vi "lv_Waveform.vi"() -> ()   [LabVIEW 2018]
panel:
  in  "位置参数":bool
  in  "时间模式":bool
  in  "还原指针":bool
  in  "鼠标拖动":bool
  in  "水平选择":bool
  in  "垂直选择":bool
  in  "点击缩小":bool
  in  "点击放大":bool
  in  "选择区域":bool
  in  "区域还原":bool
  in  "stop":bool
  out "Waveform Graph":waveform(dbl)(graph)
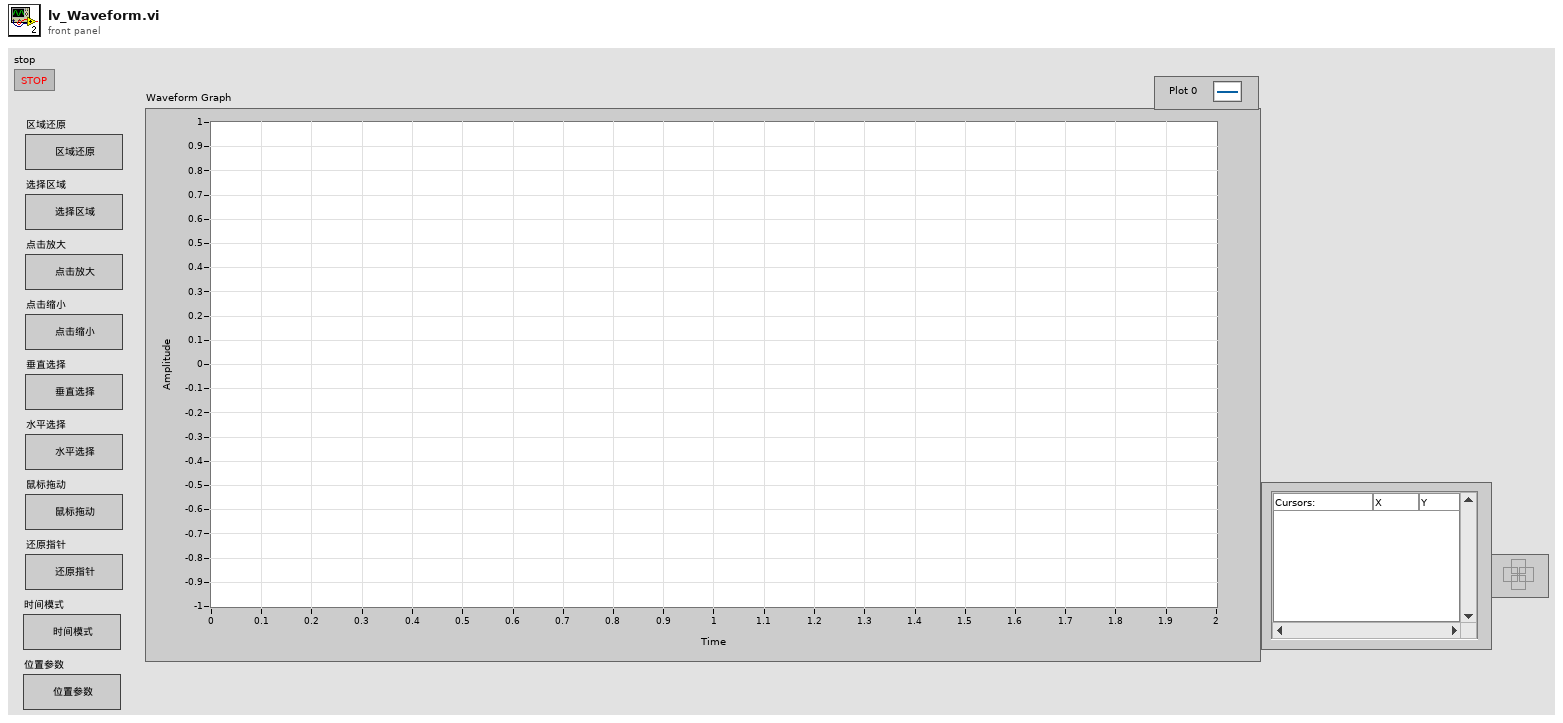
[diagram p1: front panel]
types:
  T1 = cluster{"Name":string, "Color":u32, "Style":u8, "Point Style":u8, "Name Visible":bool, "Allow Drag":bool, "Cursor Mode":u32, "Plot":i32, "Index":i32, "Position":cluster{"X":dbl, "Y":dbl}, "X Scale":u32, "Y Scale":u32, "Watch Plots":i32[], "Watch All Plots":bool, "Plot Area":i32, "Label Offset":cluster{"X":dbl, "Y":dbl}}
  T2 = cluster{"Boolean Text.Text":string, "Palette:Active Tool":i32}[]
  T3 = cluster{"Boolean Text.Text":string, "Palette:Active Tool":i32}
  T4 = typedef "LVPoint32TypeDef.ctl" = cluster{"Horizontal":i32, "Vertical":i32}
  T5 = typedef "LVCursorListTypeDef.ctl" = cluster{"Name":string, "Color":u32, "Style":u8, "Point Style":u8, "Name Visible":bool, "Allow Drag":bool, "Cursor Mode":u32, "Plot":i32, "Index":i32, "Position":cluster{"X":dbl, "Y":dbl}, "X Scale":u32, "Y Scale":u32, "Watch Plots":i32[], "Watch All Plots":bool, "Plot Area":i32, "Label Offset":cluster{"X":dbl, "Y":dbl}}[]
  T6 = typedef "LVRangeTypeDef.ctl" = cluster{"Minimum":dbl, "Maximum":dbl, "Increment":dbl, "Minor Increment":dbl, "Start":dbl}
  T7 = typedef "lveventtype.ctl" = enum32{"Null", "Timeout", "Annotation Menu Selection", "Annotation Menu Selection?", "App Instance Close", "App Instance Close?", "Autoscale Range Change", "Bookmark Info Change", "Cell Edit", "Cell Edit?", "Cursor Grab", "Cursor Grab?", "Cursor Menu Selection", "Cursor Menu Selection?", "Cursor Move", "Cursor Release", "Data Change", "Direction Change", "Display State Change", "Drag Ended", "Drag Enter", "Drag Leave", "Drag Over", "Drag Source Update", "Drag Starting", "Drag Starting?", "Drop", "Exec State Change", "Key Down", "Key Down?", "Key Repeat", "Key Repeat?", "Key Up", "Listbox Double Click", "Menu Activation?", "Menu Selection (App)", "Menu Selection? (App)", "Menu Selection (User)", "Mouse Down", "Mouse Down?", "Mouse Enter", "Mouse Leave", "Mouse Move", "Mouse Up", "Mouse Wheel", "NI Security User Change (App)", "Pane Size", "Panel Close", "Panel Close?", "Panel Resize", "Plot Attribute Change", "Scale Range Change", "Shortcut Menu Activation?", "Shortcut Menu Selection (App)", "Shortcut Menu Selection? (App)", "Shortcut Menu Selection (User)", "Tree Double Click", "Tree Drag", "Tree Drag?", "Tree Drop", "Tree Drop?", "Tree Item Close", "Tree Item Close?", "Tree Item Open", "Tree Item Open?", "User Event", "Value Change"}
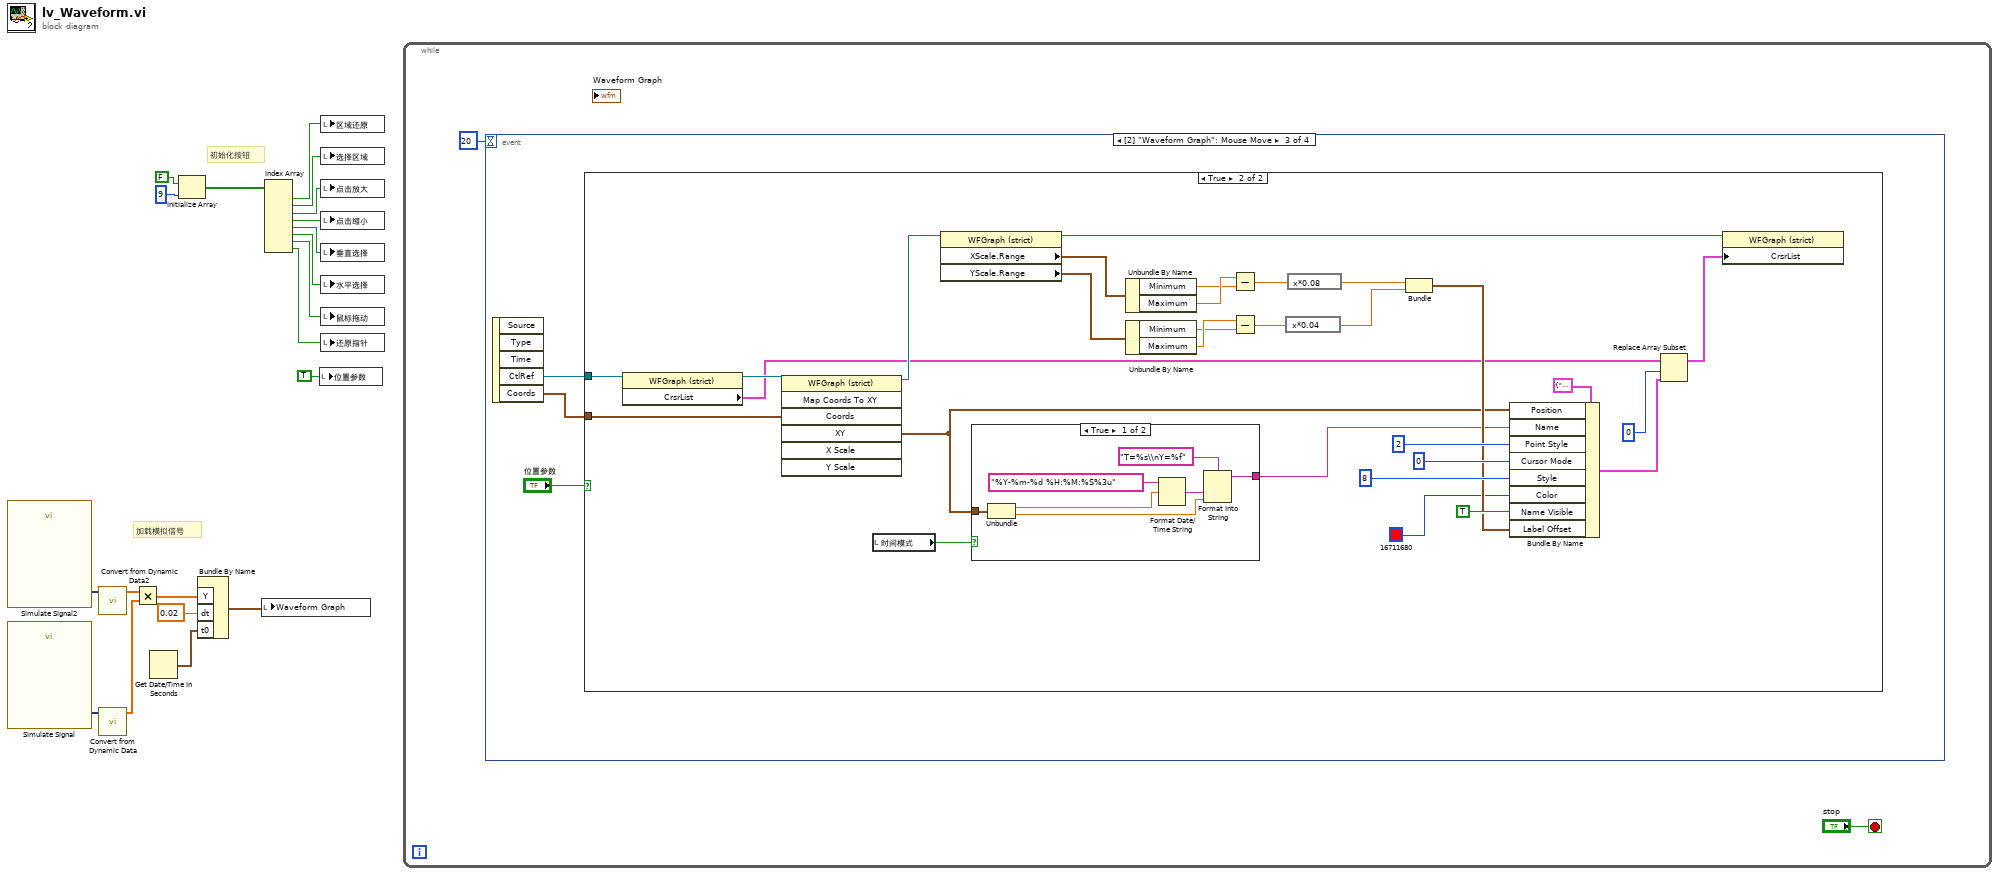
[diagram p0: block diagram]
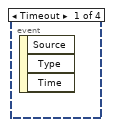
[diagram p2: hidden frame]
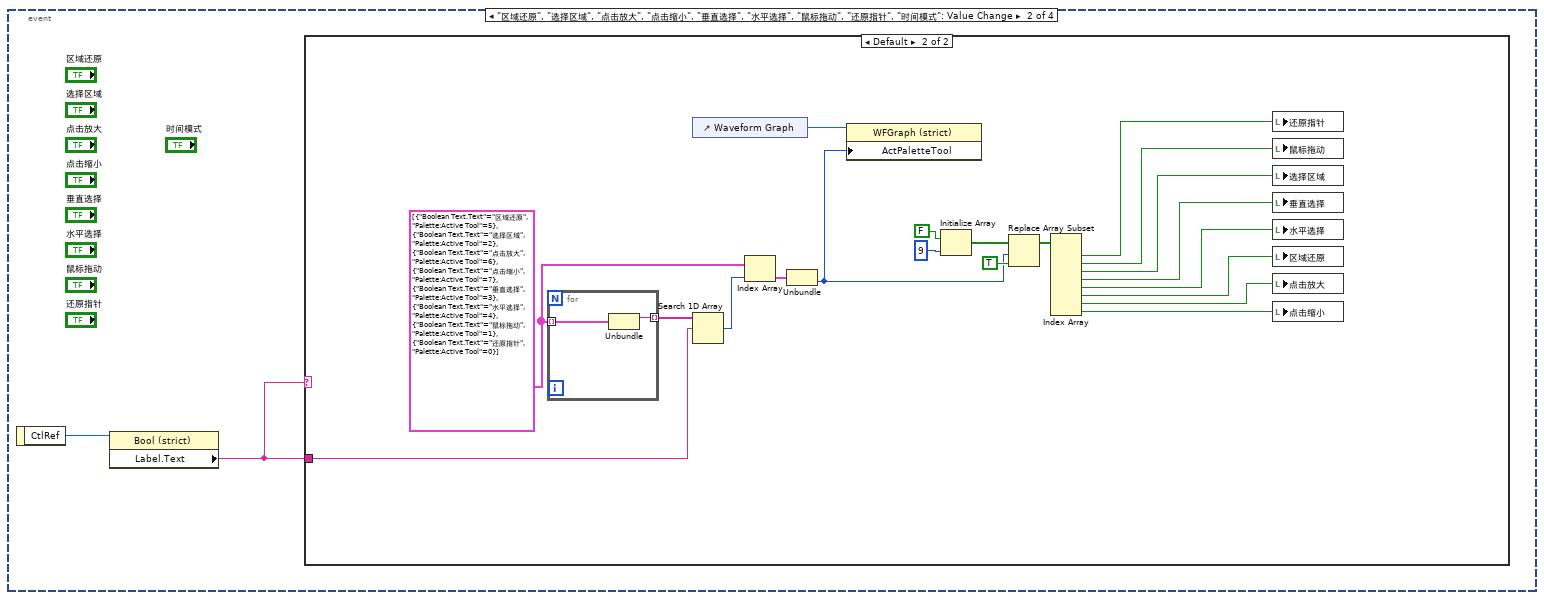
[diagram p3: hidden frame]
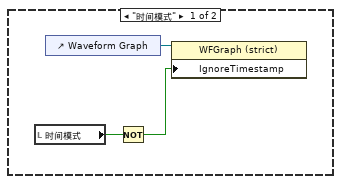
[diagram p4: hidden frame]
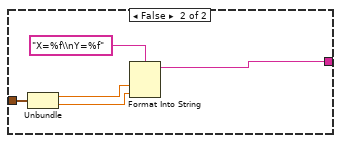
[diagram p6: hidden frame]
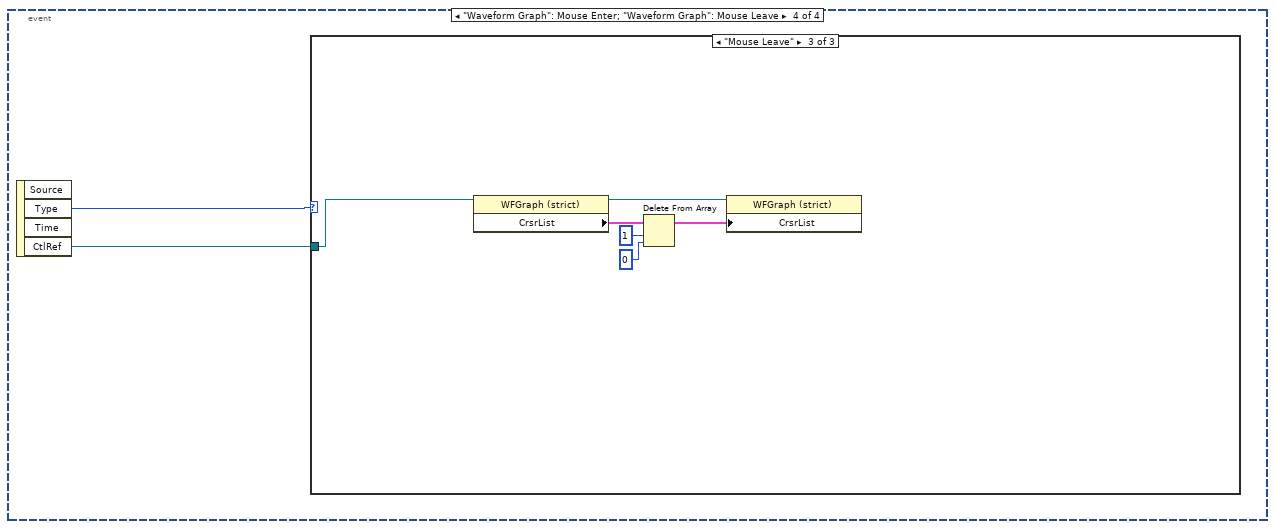
[diagram p7: hidden frame]
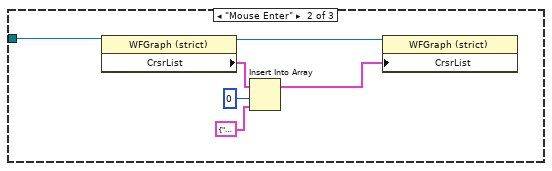
[diagram p9: hidden frame]
diagram:
  # "初始化按钮"
  # "加载模拟信号"
  n1 = call "Simulate Signal2"() -> ("Sine"=w4:dynamicdata)  [unwired: 14 in, 1 out]
  n2 = call "Simulate Signal"() -> ("Sine"=w20:dynamicdata)  [unwired: 14 in, 1 out]
  n3 = call "Convert from Dynamic Data2"("Dynamic Data Type"=w4) -> ("Array"=w3:dbl[])  [unwired: 3 in]
  n4 = call "Convert from Dynamic Data"("Dynamic Data Type"=w20) -> ("Array"=w2:dbl[])  [unwired: 3 in]
  n5 = Multiply(x=w3, y=w2) -> (x*y=w1:dbl[])
  n6 = Get Date/Time In Seconds() -> (seconds since 1Jan1904=w7:timestamp)
  n7 = Initialize Array(FALSE ("区域还原"), 9 ("dimension size")) -> (w10:bool[])
  n8 = Bundle By Name("Y"=w1, "dt"=0.02, "t0"=w7) -> (w6:waveform(dbl))  [unwired: 1 in]
  n9 = local write "Waveform Graph"(w6) -> ()
  n10 = Index Array(array=w10) -> (element #1=w13:bool, element #2=w14:bool, element #3=w15:bool, element #4=w16:bool, element #5=w17:bool, element #6=w18:bool, element #7=w19:bool, element #8=w9:bool)  [unwired: 8 in]
  n11 = local write "位置参数"(TRUE ("位置参数")) -> ()
  n12 = local write "区域还原"(w13) -> ()
  n13 = local write "选择区域"(w14) -> ()
  n14 = local write "点击放大"(w15) -> ()
  n15 = local write "点击缩小"(w16) -> ()
  n16 = local write "垂直选择"(w17) -> ()
  n17 = local write "水平选择"(w18) -> ()
  n18 = local write "鼠标拖动"(w19) -> ()
  n19 = local write "还原指针"(w9) -> ()
  n20 = while {
    stop <- "stop" stop-if-true
    n21 = event shown="[2] \"Waveform Graph\": Mouse Move" {
      selector: _ -> [_ _ _ _]
      dyn-events: _ -> [_ _ _ _]
      timeout: 20 -> [_ _ _ _]
      event Timeout {
        n22 = event-data() -> ()  [unwired: 1 in, 3 out]
      }
      event "区域还原", "选择区域", "点击放大", "点击缩小", "垂直选择", "水平选择", "鼠标拖动", "还原指针", "时间模式": Value Change {
        n23 = event-data() -> ("CtlRef"=w24:refnum<vi>)  [unwired: 1 in]
        n24 = property class="Bool (strict)"(reference=w24) -> ("Label.Text"=w23:string)  [unwired: 1 in, 2 out]
        n25 = case shown="Default" w23 {
          tunnel: w23 -> [_ w46]
          frame "时间模式" {
            n26 = local read "时间模式"() -> (w26:bool)
            n27 = control-ref of="Waveform Graph"() -> (w27:refnum<vi>)
            n28 = Not(x=w26) -> (.not. x?=w25:bool)
            n29 = property on="Property Node" class="WFGraph (strict)"(reference=w27, "IgnoreTimestamp"=w25) -> ()  [unwired: 1 in, 2 out]
          }
          frame Default {
            w43 = T2 [{"Boolean Text.Text"="区域还原", "Palette:Active Tool"=5}, {"Boolean Text.Text"="选择区域", "Palette:Active Tool"=2}, {"Boolean Text.Text"="点击放大", "Palette:Active Tool"=6}, {"Boolean Text.Text"="点击缩小", "Palette:Active Tool"=7}, {"Boolean Text.Text"="垂直选择", "Palette:Active Tool"=3}, {"Boolean Text.Text"="水平选择", "Palette:Active Tool"=4}, {"Boolean Text.Text"="鼠标拖动", "Palette:Active Tool"=1}, {"Boolean Text.Text"="还原指针", "Palette:Active Tool"=0}]
            n30 = for {
              tunnel: w43 -> [w49] mode=indexing
              tunnel: [w48] -> w47 mode=indexing
              n31 = Unbundle(w49) -> ("Boolean Text.Text"=w48:string)  [unwired: 1 out]
            }
            n32 = control-ref of="Waveform Graph"() -> (w36:refnum<vi>)
            n33 = Search 1D Array(1D array=w47, element=w46) -> (index of element=w44:i32)  [unwired: 1 in]
            n34 = Index Array(array=w43, index=w44) -> (element=w45:T3)
            n35 = Unbundle(w45) -> ("Palette:Active Tool"=w37:i32)  [unwired: 1 out]
            n36 = property on="Property Node" class="WFGraph (strict)"(reference=w36, "ActPaletteTool"=w37) -> ()  [unwired: 1 in, 2 out]
            n37 = Initialize Array(FALSE ("区域还原"), 9 ("dimension size")) -> (w41:bool[])
            n38 = Replace Array Subset(array=w41, new element=TRUE ("new element/subarray"), index=w37) -> (w38:bool[])
            n39 = Index Array(array=w38) -> (element #1=w28:bool, element #2=w29:bool, element #3=w34:bool, element #4=w31:bool, element #5=w30:bool, element #6=w35:bool, element #7=w33:bool, element #8=w32:bool)  [unwired: 8 in]
            n40 = local write "还原指针"(w28) -> ()
            n41 = local write "鼠标拖动"(w29) -> ()
            n42 = local write "选择区域"(w34) -> ()
            n43 = local write "垂直选择"(w31) -> ()
            n44 = local write "水平选择"(w30) -> ()
            n45 = local write "区域还原"(w35) -> ()
            n46 = local write "点击放大"(w33) -> ()
            n47 = local write "点击缩小"(w32) -> ()
          }
        }
      }
      event "Waveform Graph": Mouse Move {
        n48 = event-data() -> ("CtlRef"=w52:refnum<vi>, "Coords"=w51:T4)  [unwired: 1 in, 3 out]
        n49 = case shown="True" "位置参数" {
          tunnel: w52 -> [_ w81]
          tunnel: w51 -> [_ w80]
          frame False {
          }
          frame True {
            n50 = property on="Property Node" class="WFGraph (strict)"(reference=w81) -> (reference out=w79:refnum<vi>, "CrsrList"=w57:T5)  [unwired: 1 in, 1 out]
            n51 = invoke on="Invoke Node" class="WFGraph (strict)" method="Map Coords To XY"(reference=w79, "Coords"=w80) -> (reference out=w68:refnum<vi>, "XY"=w61:cluster{"X":dbl, "Y":dbl})  [unwired: 5 in, 5 out]
            n52 = local read "时间模式"() -> (w53:bool)
            n53 = property on="Property Node" class="WFGraph (strict)"(reference=w68) -> (reference out=w59:refnum<vi>, "XScale.Range"=w74:T6, "YScale.Range"=w71:T6)  [unwired: 1 in, 1 out]
            n54 = case shown="True" w53 {
              tunnel: w61 -> [w88 w92]
              tunnel: [w86 w89] -> w60
              frame True {
                n55 = Unbundle(w88) -> ("X"=w85:dbl, "Y"=w83:dbl)
                n56 = Format Date/Time String(time format string (%c)="%Y-%m-%d %H:%M:%S%3u" ("format string"), seconds (now)=w85) -> (date/time string=w84:string)  [unwired: 1 in]
                n57 = Format Into String(format string="T=%s\\nY=%f", w84, w83) -> (resulting string=w86:string)  [unwired: 2 in, 1 out]
              }
              frame False {
                n58 = Unbundle(w92) -> ("X"=w91:dbl, "Y"=w90:dbl)
                n59 = Format Into String(format string="X=%f\\nY=%f", w91, w90) -> (resulting string=w89:string)  [unwired: 2 in, 1 out]
              }
            }
            n60 = Unbundle By Name(w74) -> ("Minimum"=w72:dbl, "Maximum"=w73:dbl)
            n61 = Unbundle By Name(w71) -> ("Minimum"=w69:dbl, "Maximum"=w70:dbl)
            n62 = Subtract(x=w73, y=w72) -> (x-y=w75:dbl)
            n63 = Subtract(x=w70, y=w69) -> (x-y=w76:dbl)
            n64 = expression code="x*0.04"(w76) -> (w78:dbl)
            n65 = expression code="x*0.08"(w75) -> (w77:dbl)
            n66 = Bundle(w77, w78) -> (w62:cluster{dbl, dbl})  [unwired: 1 in]
            n67 = Bundle By Name(cluster=T1 {"Name"="", "Color"=0, "Style"=0, "Point Style"=0, "Name Visible"=FALSE, "Allow Drag"=FALSE, "Cursor Mode"=0, "Plot"=0, "Index"=0, "Position"={"X"=0.0, "Y"=0.0}, "X Scale"=0, "Y Scale"=0, "Watch Plots"=[], "Watch All Plots"=FALSE, "Plot Area"=0, "Label Offset"={"X"=0.0, "Y"=0.0}}, "Position"=w61, "Name"=w60, "Point Style"=u8 2, "Cursor Mode"=u32 0, "Style"=u8 8 ("M2Style 2"), "Color"=u32 16711680 ("游标颜色"), "Name Visible"=TRUE, "Label Offset"=w62) -> (w56:T1)
            n68 = Replace Array Subset "Replace Array Subset"(array=w57, new element=w56, index=0) -> (w55:T5)
            n69 = property on="Property Node" class="WFGraph (strict)"(reference=w59, "CrsrList"=w55) -> ()  [unwired: 1 in, 2 out]
          }
        }
      }
      event "Waveform Graph": Mouse Enter; "Waveform Graph": Mouse Leave {
        n70 = event-data() -> ("Type"=w95:T7, "CtlRef"=w94:refnum<vi>)  [unwired: 1 in, 2 out]
        n71 = case shown="\"Mouse Leave\"" w95 {
          tunnel: w94 -> [_ w96 w102]
          frame Default {
          }
          frame "Mouse Enter" {
            n72 = property on="Property Node" class="WFGraph (strict)"(reference=w96) -> (reference out=w101:refnum<vi>, "CrsrList"=w100:T5)  [unwired: 1 in, 1 out]
            n73 = Insert Into Array "Insert Into Array"(array=w100, index=0, new element=T1 {"Name"="", "Color"=0, "Style"=0, "Point Style"=0, "Name Visible"=FALSE, "Allow Drag"=FALSE, "Cursor Mode"=0, "Plot"=0, "Index"=0, "Position"={"X"=0.0, "Y"=0.0}, "X Scale"=0, "Y Scale"=0, "Watch Plots"=[], "Watch All Plots"=FALSE, "Plot Area"=0, "Label Offset"={"X"=0.0, "Y"=0.0}}) -> (w99:T5)
            n74 = property on="Property Node" class="WFGraph (strict)"(reference=w101, "CrsrList"=w99) -> ()  [unwired: 1 in, 2 out]
          }
          frame "Mouse Leave" {
            n75 = property on="Property Node" class="WFGraph (strict)"(reference=w102) -> (reference out=w105:refnum<vi>, "CrsrList"=w106:T5)  [unwired: 1 in, 1 out]
            n76 = Delete From Array(array=w106, length=1, index=0) -> (array with subset deleted=w107:T5)  [unwired: 1 out]
            n77 = property on="Property Node" class="WFGraph (strict)"(reference=w105, "CrsrList"=w107) -> ()  [unwired: 1 in, 2 out]
          }
        }
      }
    }
  }
